vi "Send Start-Stop Message.vi"(6 "Start(T)/Stop(F)":bool, 8 "Error In":errorcluster, 9 "Version number":string, 10 "Software Name":string, 11 "Notebook Queue":refnum<queue>) -> (0 "Error Out":errorcluster)   [LabVIEW 2019, in "Notebook.lvlib"]
uses:
  Notebook.lvlib
  Notebook Action Q Element.ctl
  Notebook Action List.ctl
  Rich Text Box/Rich Text Box.lvlib
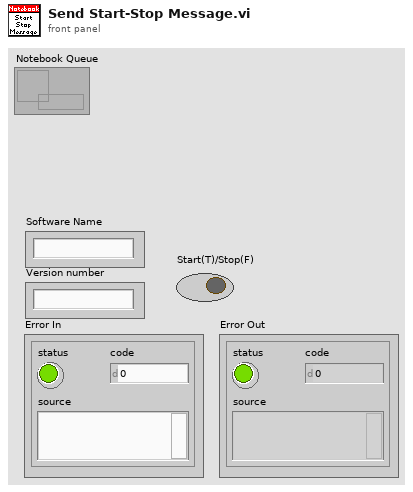
[diagram p1: front panel]
types:
  T1 = typedef "Rich Text Box.lvlib/Text Formatting.ctl" = cluster{"Font":string, "Text Color":T2, "Text Background Color":T2, "Text Style":enum16{"Regular", "Bold", "Italic", "Underline", "Strikeout"}, "Font Size (Points)":dbl, "Text Alignment":i32}
  T2 = typedef "Rich Text Box.lvlib/Text Colors.ctl" = enum16{"Unchanged", "Black", "Blue", "Brown", "Gray", "Green", "Orange", "Pink", "Red", "White"}
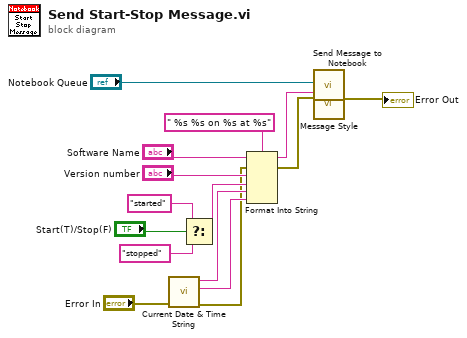
[diagram p0: block diagram]
diagram:
  n1 = call "Current Date & Time String.vi"("Error In"="Error In") -> ("Error Out"=w5:errorcluster, "time string"=w8:string, "date string"=w9:string)  [unwired: 8 in]
  n2 = Select(t="started" ("Version number"), s="Start(T)/Stop(F)", f="stopped" ("Version number")) -> (s? t:f=w12:string)
  n3 = Format Into String(format string=" %s %s on %s at %s", initial string="Software Name", error in=w5, "Version number", w12, w9, w8) -> (resulting string=w11:string, error out=w4:errorcluster)
  n4 = call "Message Style.vi"() -> ("Message Formatting"=w10:T1)
  n5 = call "Send Message to Notebook.vi"("Notebook Queue"="Notebook Queue", "Message"=w11, "Error In"=w4, "Text Formatting"=w10) -> ("Error Out"=→"Error Out":errorcluster)  [unwired: 15 in]
